vi "Kitchen Timer.vi"() -> ()   [LabVIEW 2017]
panel:
  in  "Timer (sec)":i32(knob) scale=0.0..60.0
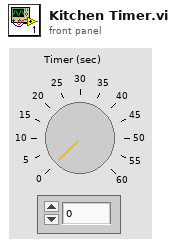
[diagram p1: front panel]
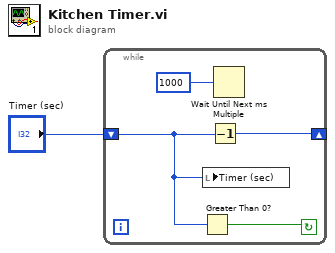
[diagram p0: block diagram]
diagram:
  n1 = while {
    shift-right: [w5] -> _
    shift-left: "Timer (sec)" -> [w4]
    stop <- w3 continue-if-true
    n2 = Greater Than 0?(x=w4) -> (x > 0?=w3:bool)
    n3 = local write "Timer (sec)"(w4) -> ()
    n4 = Decrement(x=w4) -> (x-1=w5:i32)
    n5 = Wait Until Next ms Multiple(millisecond multiple=1000) -> ()  [unwired: 1 out]
  }
